vi "Module - Template.vi"() -> ()   [LabVIEW 2020]
panel:
  out "error out":errorcluster
  in  "error in (no error)":errorcluster
types:
  T1 = enum16{"Init module", "Register event", "Idle", "Process", "Unregister event", "Close module"}
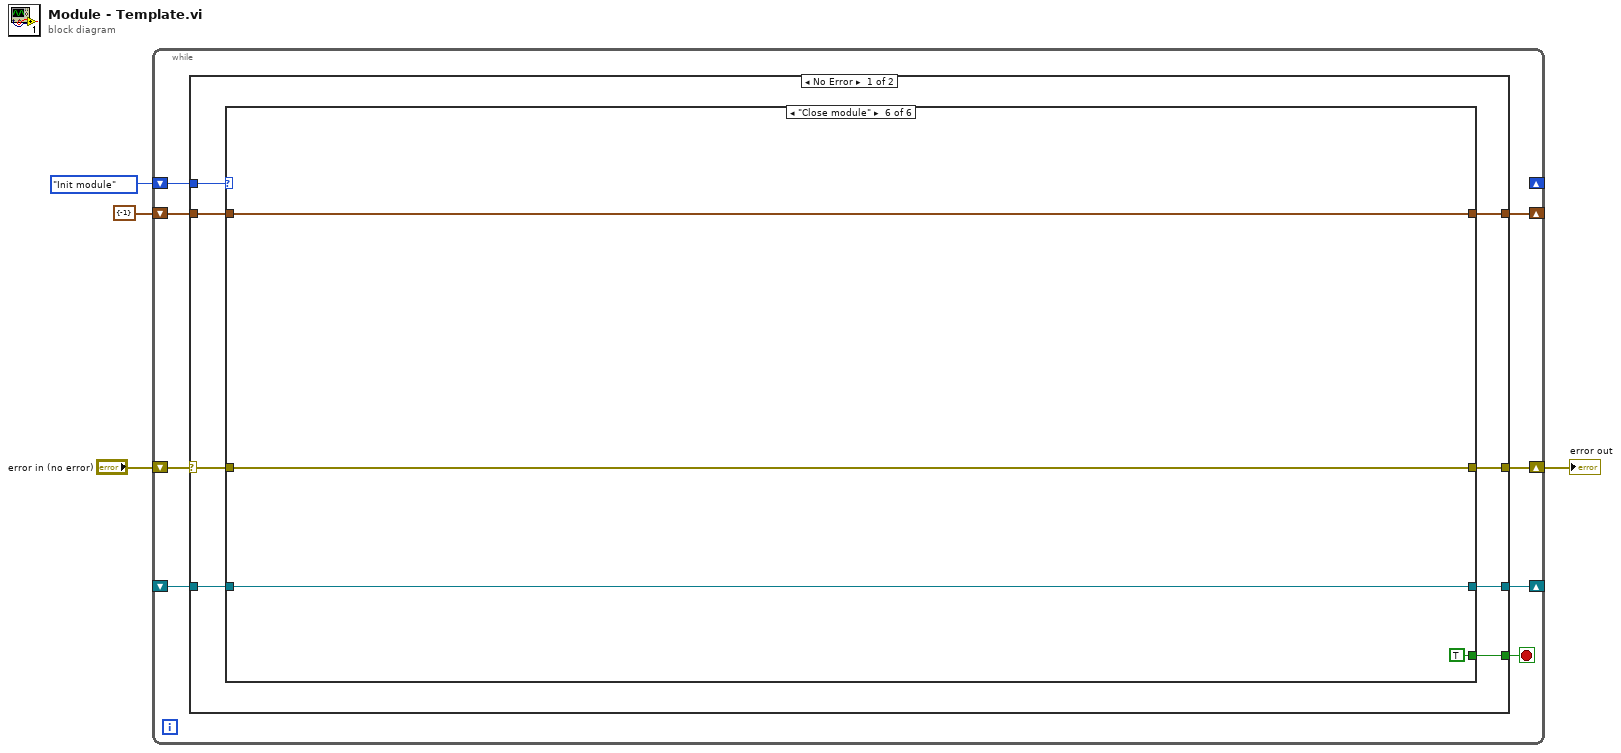
[diagram p0: block diagram]
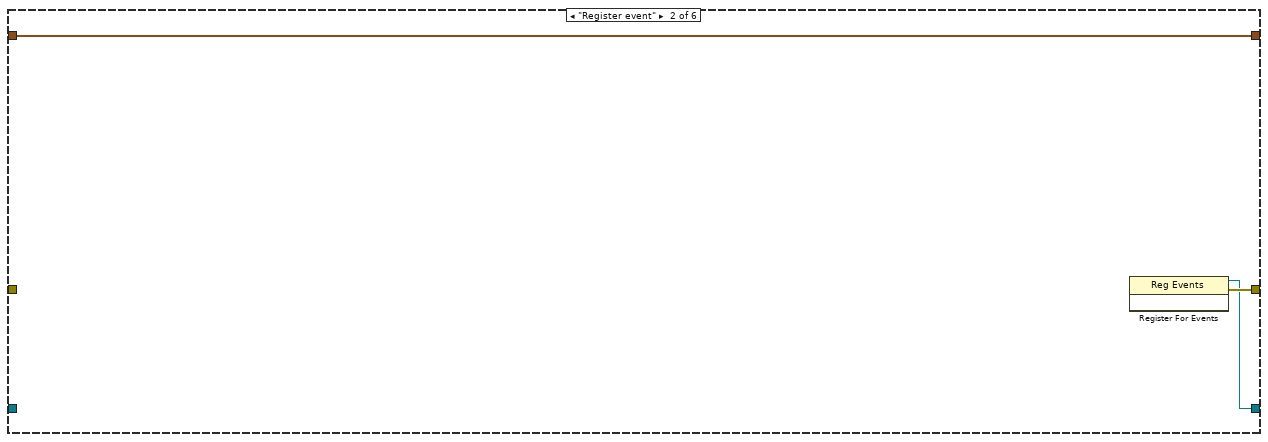
[diagram p3: hidden frame]
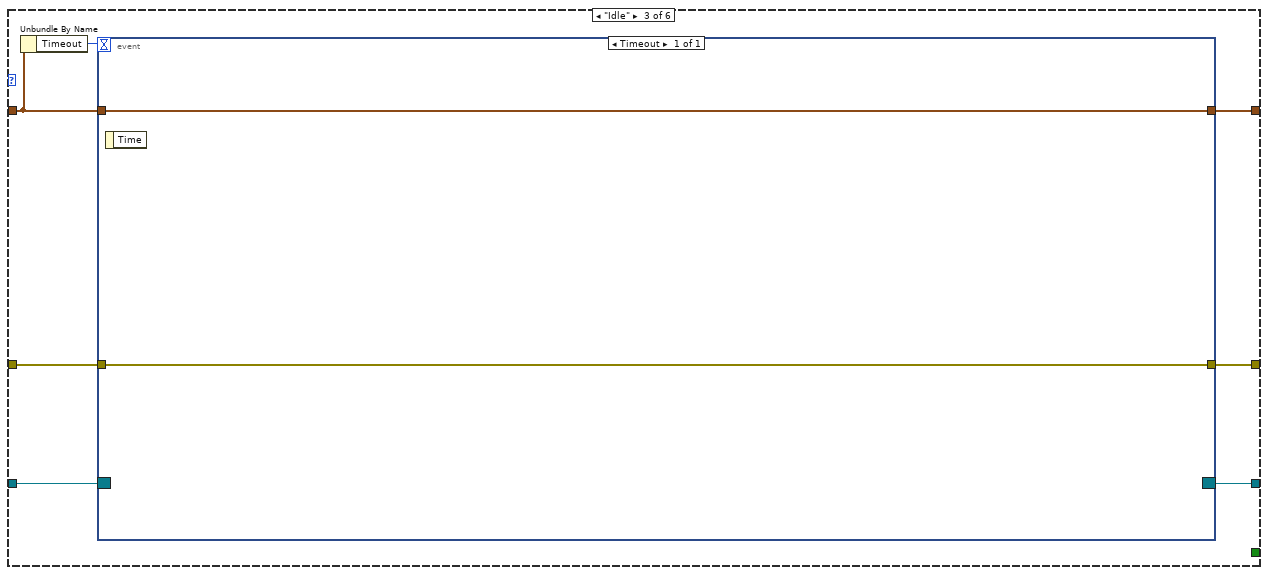
[diagram p4: hidden frame]
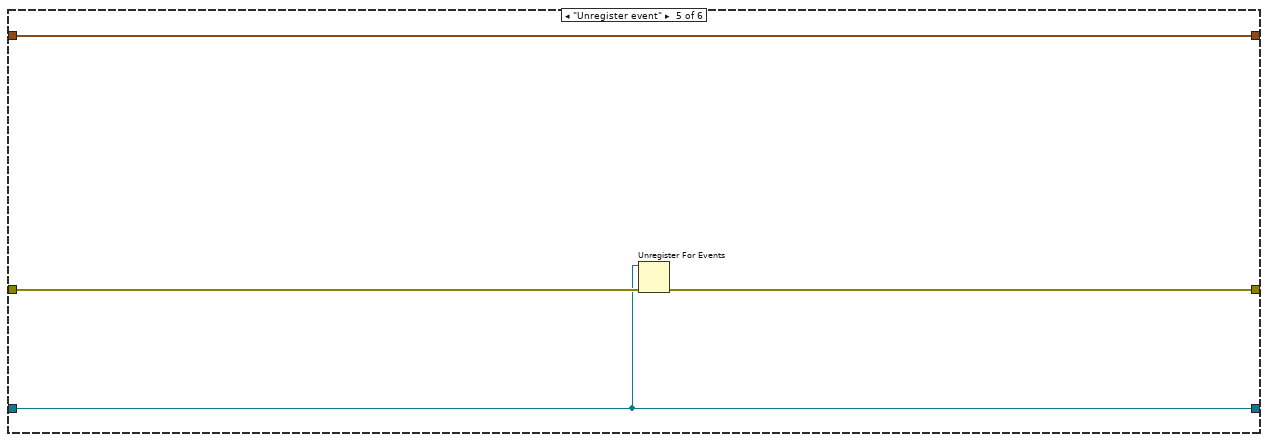
[diagram p6: hidden frame]
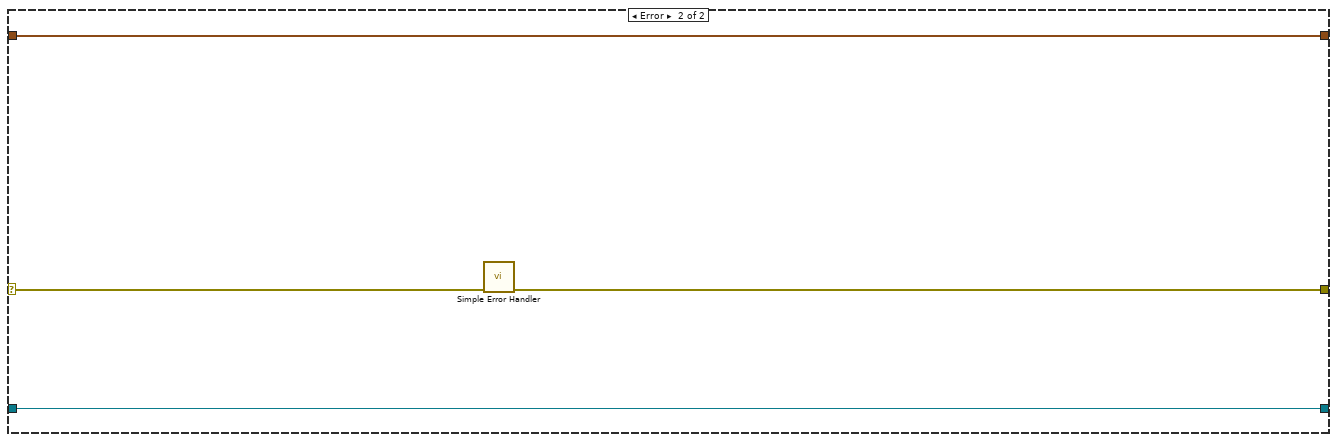
[diagram p7: hidden frame]
diagram:
  n1 = while {
    shift-right: [w10] -> w3
    shift-left: "error in (no error)" -> [w12]
    shift-right: _ -> [_]
    shift-left: T1."Init module" -> [w11]
    shift-right: [w9] -> _
    shift-left: _ -> [w8]
    shift-right: [w6] -> _
    shift-left: cluster{"Timeout":i32} {"Timeout"=-1} -> [w7]
    stop <- w5 stop-if-true
    n2 = case shown="No Error" w12 {
      selector: w12 -> [w19 w50]
      tunnel: w11 -> [w20 _]
      tunnel: [w18 w49] -> w10
      tunnel: [w17 w48] -> w9
      tunnel: w8 -> [w16 w48]
      tunnel: w7 -> [w15 w47]
      tunnel: [w14 w47] -> w6
      tunnel: [w13 _] -> w5
      frame No Error {
        n3 = case shown="\"Close module\"" w20 {
          tunnel: w19 -> [w23 _ w30 w38 w41 w46]
          tunnel: [w23 w26 w27 w38 w40 w46] -> w18
          tunnel: [w22 w25 w28 w37 w39 w45] -> w17
          tunnel: w16 -> [w22 _ w29 w37 w39 w45]
          tunnel: w15 -> [w21 w24 w32 w36 w42 w44]
          tunnel: [w21 w24 w31 w36 w42 w44] -> w14
          tunnel: [_ _ _ _ _ TRUE] -> w13
          frame "Init module", Default {
          }
          frame "Register event" {
            n4 = register-events() -> (reference out=w25:refnum<event-registration>, error out=w26:errorcluster)  [unwired: 3 in]
          }
          frame "Idle" {
            n5 = Unbundle By Name(w32) -> ("Timeout"=w33:i32)
            n6 = event shown="[0] Timeout" {
              selector: w29 -> [_]
              dyn-events: [_] -> w28
              timeout: w33 -> [_]
              tunnel: w32 -> [w35]
              tunnel: [w35] -> w31
              tunnel: w30 -> [w34]
              tunnel: [w34] -> w27
              event Timeout {
                n7 = event-data() -> ()  [unwired: 1 in, 1 out]
              }
            }
          }
          frame "Process" {
          }
          frame "Unregister event" {
            n8 = Unregister For Events(event registration refnum=w39, error in=w41) -> (error out=w40:errorcluster)
          }
          frame "Close module" {
          }
        }
      }
      frame Error {
        n9 = call <vilib>:"Simple Error Handler.vi"("error in (no error)"=w50) -> ("error out"=w49:errorcluster)  [unwired: 4 in, 4 out]
      }
    }
  }
  "error out" <- w3
